vi "Chi-Squared Random.vi"(6 "seed":i32=-1, 7 "reset":bool, 10 "k":i32=1, 11 "samples":i32=128) -> (0 "error":i32, 3 "chi-squared random data":dbl[](array[numeric]))   [LabVIEW 2010, in "NI_Gmath.lvlib"]
doc: "Generates random values from a variate X, where X describes the selected distribution type. You must manually select the polymorphic instance to use."
uses:
  NI_Gmath.lvlib
panel:
  # "Chi-Squared Random"
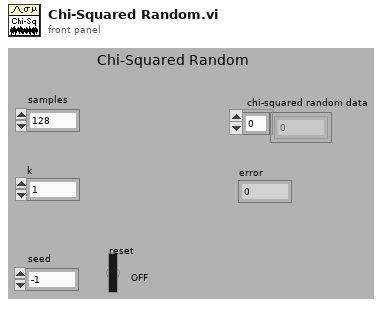
[diagram p1: front panel]
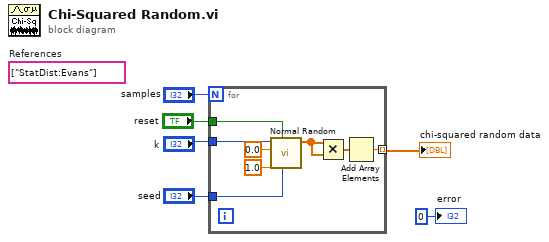
[diagram p0: block diagram]
diagram:
  (unwired) string[] ["StatDist:Evans"]  # References
  n1 = for {
    N: "samples" -> [_]
    tunnel: "k" -> [w10]
    tunnel: "seed" -> [w14]
    tunnel: [w13] -> w2 mode=indexing
    tunnel: "reset" -> [w7]
    n2 = call "Normal Random.vi"("seed"=w14, "reset"=w7, "std"=1.0, "mean"=0.0, "samples"=w10) -> ("normal random data"=w9:dbl[])  [unwired: 5 in, 1 out]
    n3 = Multiply(x=w9, y=w9) -> (x*y=w8:dbl[])
    n4 = Add Array Elements(numeric array=w8) -> (sum=w13:dbl)
  }
  "chi-squared random data" <- w2
  "error" <- 0 ("error")
